vi "Configure State File.vi"(7 "Auto Recall (T: Enable)":bool=TRUE, 8 "error in (no error)":errorcluster, 9 "File Name ()":string, 10 "State File Operation (0: Load State File)":i32(ring) items=["Load State File", "Store State File", "Recall State File"], 11 "VISA resource name":refnum<visa-resource-name>) -> (0 "error out":errorcluster, 3 "VISA resource name out":refnum<visa-resource-name>)   [LabVIEW 2013, in "Agilent 3446X Series.lvlib"]
doc: "Configures the state file."
uses:
  Agilent 3446X Series.lvlib
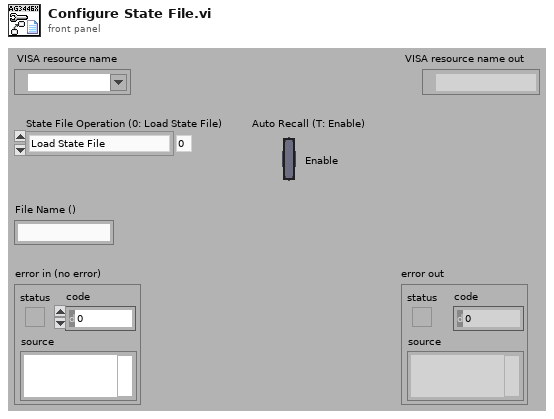
[diagram p1: front panel]
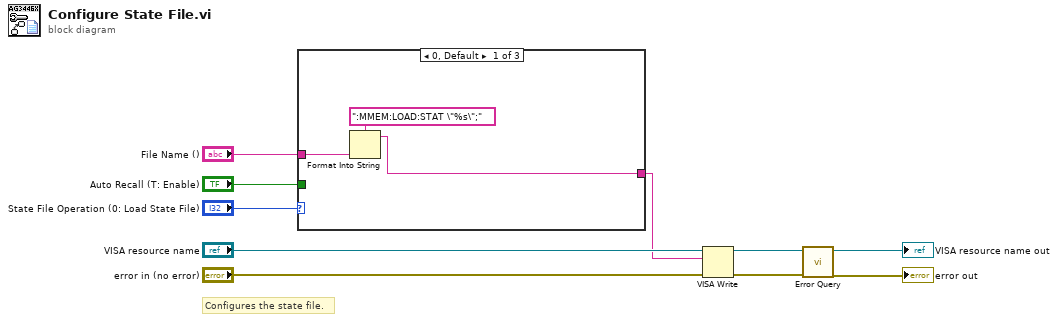
[diagram p0: block diagram]
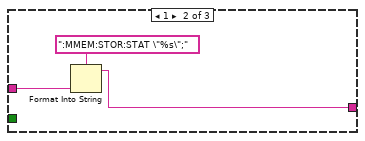
[diagram p2: hidden frame]
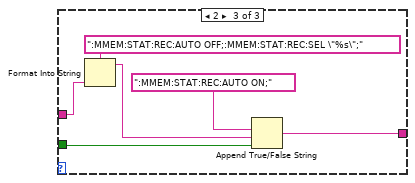
[diagram p3: hidden frame]
diagram:
  # "Configures the state file."
  n1 = case shown="0, Default" "State File Operation (0: Load State File)" {
    tunnel: "File Name ()" -> [w12 w16 w17]
    tunnel: [w11 w14 w18] -> w1
    tunnel: "Auto Recall (T: Enable)" -> [_ _ w21]
    frame 0, Default {
      n2 = Format Into String(format string=":MMEM:LOAD:STAT \"%s\";", w12) -> (resulting string=w11:string)  [unwired: 2 in, 1 out]
    }
    frame 1 {
      n3 = Format Into String(format string=":MMEM:STOR:STAT \"%s\";", w16) -> (resulting string=w14:string)  [unwired: 2 in, 1 out]
    }
    frame 2 {
      n4 = Format Into String(format string=":MMEM:STAT:REC:AUTO OFF;:MMEM:STAT:REC:SEL \"%s\";", w17) -> (resulting string=w19:string)  [unwired: 2 in, 1 out]
      n5 = Append True/False String(1:w21, 2:w19, 3:":MMEM:STAT:REC:AUTO ON;") -> (0:w18:string)  [unwired: 1 out]
    }
  }
  n6 = VISA Write(VISA resource name="VISA resource name", write buffer=w1, error in (no error)="error in (no error)") -> (VISA resource name out=w8:refnum<visa-resource-name>, error out=w7:errorcluster)  [unwired: 1 out]
  n7 = call "Error Query.vi"("error in (no error)"=w7, "VISA resource name"=w8) -> ("error out"=→"error out":errorcluster, "VISA resource name out"=→"VISA resource name out":refnum<visa-resource-name>)  [unwired: 8 out]
